vi "ErrorLoop.vi"(8 "Error In":errorcluster, 11 "Message Queues":T1) -> (0 "Error Out":errorcluster)   [LabVIEW 2017, in "Client.lvlib" / "ClientErrorHandler.lvlib"]
doc: "This Loop receives all errors and warnings coming from any other loop. It then validates if the error is critical, and if yes, it stops the Application by sending a UserEvent to the EHL.\nThis Loop also logs all Errors to a textfile."
uses:
  ClientErrorHandler.lvlib
  Error Cluster From Error Code.vi
  Error Ring.xnode
  Message Queue.lvlib
  ClientLogger.lvlib
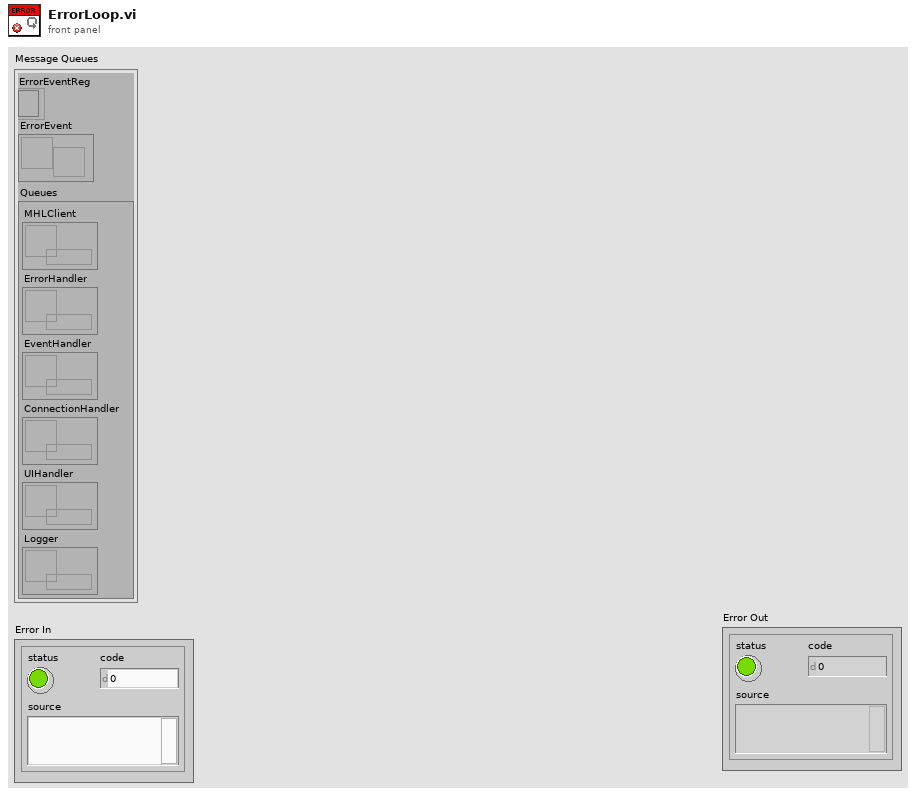
[diagram p1: front panel]
types:
  T1 = cluster{"ErrorEventReg":refnum<event-registration>, "ErrorEvent":refnum<user-event>, "Queues":cluster{"MHLClient":refnum<queue>, "ErrorHandler":refnum<queue>, "EventHandler":refnum<queue>, "ConnectionHandler":refnum<queue>, "UIHandler":refnum<queue>, "Logger":refnum<queue>}}
  T2 = cluster{"ErrorLoopInitData":cluster{"ErrorsToIgnore":i32[]}}
  T3 = cluster{"ClientTimeout (s)":u32, "LogPath":path, "ErrorsToIgnore":i32[], "OracleData":cluster{"DBname":string, "User":string, "Password":string}}
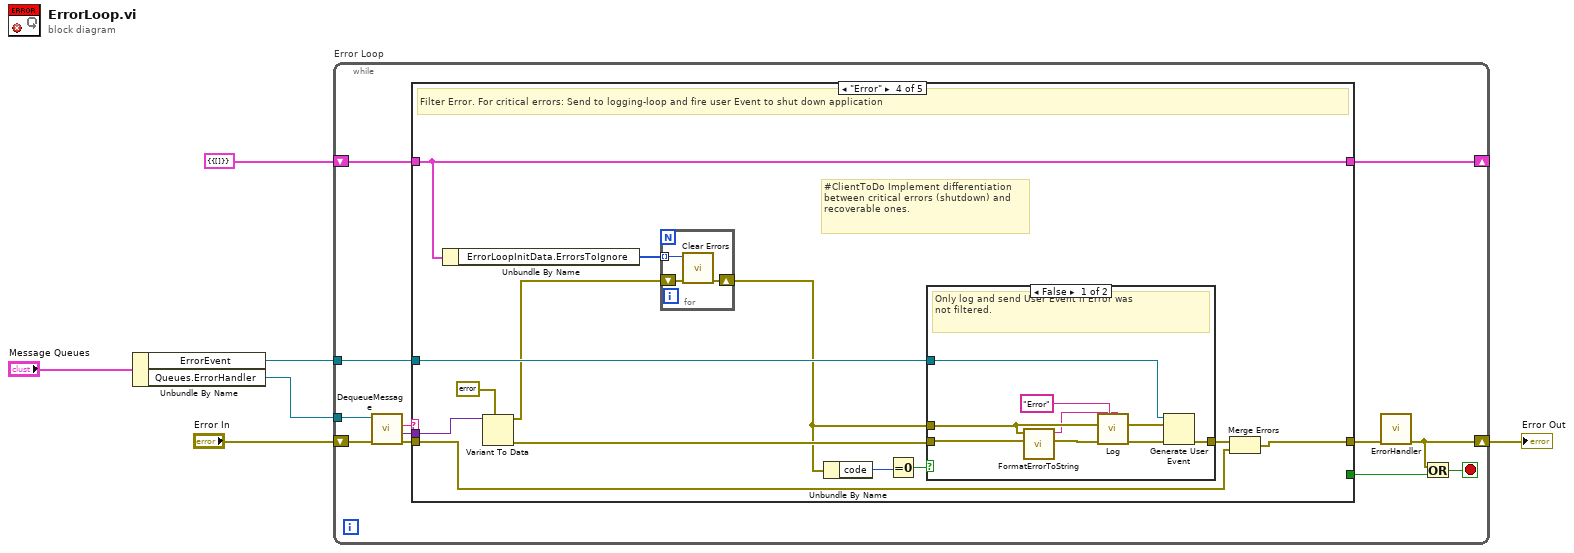
[diagram p0: block diagram]
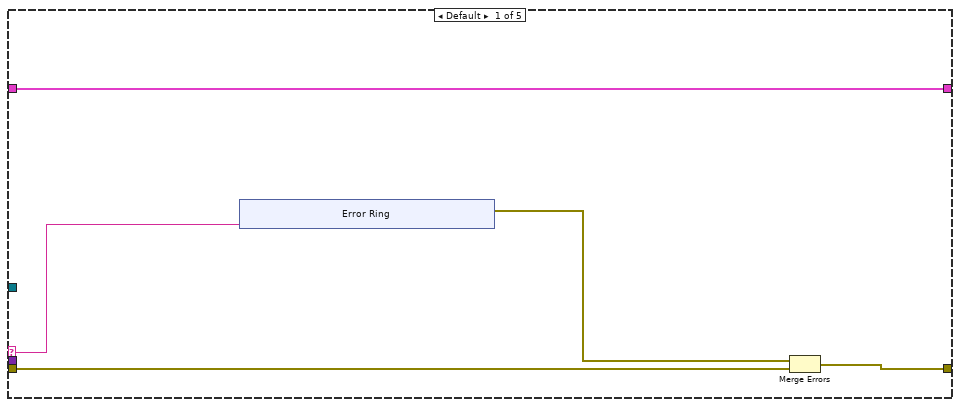
[diagram p2: hidden frame]
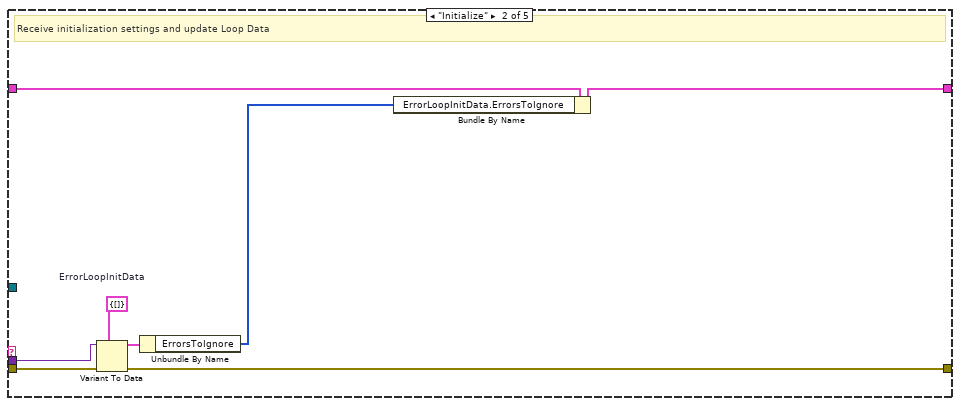
[diagram p3: hidden frame]
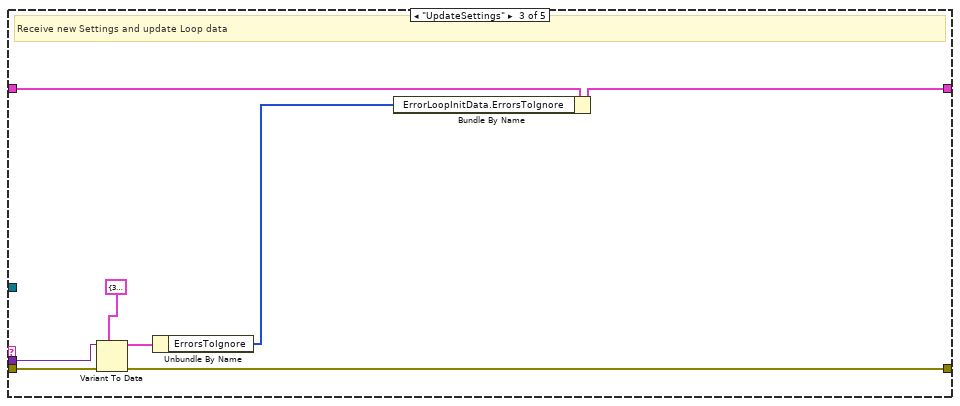
[diagram p4: hidden frame]
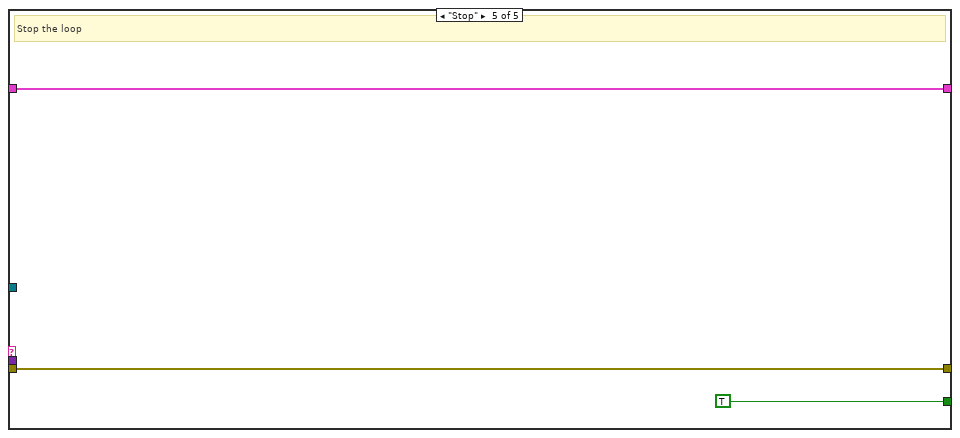
[diagram p6: hidden frame]
diagram:
  n1 = Unbundle By Name("Message Queues") -> ("ErrorEvent"=w3:refnum<user-event>, "Queues.ErrorHandler"=w4:refnum<queue>)
  n2 = while "Error Loop" {
    shift-right: [w7] -> w5
    shift-left: "Error In" -> [w18]
    tunnel: w4 -> [w16]
    tunnel: w3 -> [w11]
    shift-right: [w9] -> _
    shift-left: T2 {"ErrorLoopInitData"={"ErrorsToIgnore"=[]}} ("ErrorLoopData") -> [w10]
    stop <- w8 stop-if-true
    n3 = call "DequeueMessage.vi"("error in (no error)"=w18, "Message Queue"=w16) -> ("error out"=w17:errorcluster, "Message Data"=w14:variant, "Message"=w15:string)  [unwired: 5 in, 2 out]
    n4 = case shown="\"Error\"" w15 {
      selector: w15 -> [w20 _ _ _ _]
      tunnel: [w22 w37 w45 w55 w74] -> w12
      tunnel: w17 -> [w23 w38 w46 w53 w74]
      tunnel: w14 -> [_ w36 w44 w57 _]
      tunnel: [_ _ _ _ TRUE] -> w13
      tunnel: w11 -> [_ _ _ w58 _]
      tunnel: w10 -> [w19 w35 w42 w48 w72]
      tunnel: [w19 w34 w41 w48 w72] -> w9
      frame Default {
        n5 = xnode "Error Ring"("parameter 0"=w20) -> ("error out"=w21:errorcluster)
        n6 = Merge Errors(w21, w23) -> (w22:errorcluster)
      }
      frame "Initialize" {
        w33 = cluster{"ErrorsToIgnore":i32[]} {"ErrorsToIgnore"=[]}  # ErrorLoopInitData
        # "Receive initialization settings and update Loop Data"
        n7 = Variant To Data(error in=w38, type=w33, Variant=w36) -> (data=w32:cluster{"ErrorsToIgnore":i32[]}, error out=w37:errorcluster)
        n8 = Unbundle By Name(w32) -> ("ErrorsToIgnore"=w31:i32[])
        n9 = Bundle By Name(cluster=w35, "ErrorLoopInitData.ErrorsToIgnore"=w31) -> (w34:T2)
      }
      frame "UpdateSettings" {
        # "Receive new Settings and update Loop data"
        n10 = Variant To Data(error in=w46, type=T3 {"ClientTimeout (s)"=30, "LogPath"=path "C:/Users/jgoebel/Documents/GitHub/AEDashboard/ServerLib/Data/ServerLog.tdms", "ErrorsToIgnore"=[], "OracleData"={"DBname"="", "User"="", "Password"=""}} ("ServerINI"), Variant=w44) -> (data=w40:T3, error out=w45:errorcluster)
        n11 = Unbundle By Name(w40) -> ("ErrorsToIgnore"=w39:i32[])
        n12 = Bundle By Name(cluster=w42, "ErrorLoopInitData.ErrorsToIgnore"=w39) -> (w41:T2)
      }
      frame "Error" {
        # "#ClientToDo Implement differentiation between critical errors (shutdown) and recoverable ones."
        # "Filter Error. For critical errors: Send to logging-loop and fire user Event to shut down application"
        n13 = Unbundle By Name(w48) -> ("ErrorLoopInitData.ErrorsToIgnore"=w47:i32[])
        n14 = Variant To Data(type=errorcluster {"status"=FALSE, "code"=0, "source"=""} ("error constant"), Variant=w57) -> (data=w52:errorcluster, error out=w54:errorcluster)  [unwired: 1 in]
        n15 = for {
          shift-right: [w70] -> w51
          shift-left: w52 -> [w71]
          tunnel: w47 -> [w69] mode=indexing
          n16 = call "Clear Errors.vi"("error in (no error)"=w71, "specific error code to clear (0: all)"=w69) -> ("error out"=w70:errorcluster)  [unwired: 4 in, 1 out]
        }
        n17 = Unbundle By Name(w51) -> ("code"=w50:i32)
        n18 = Equal To 0?(x=w50) -> (x = 0?=w49:bool)
        n19 = case shown="False" w49 {
          tunnel: [w66 w68] -> w59
          tunnel: w58 -> [w64 _]
          tunnel: w54 -> [w65 w68]
          tunnel: w51 -> [w67 _]
          frame False {
            # "Only log and send User Event if Error was\nnot filtered."
            n20 = call "FormatErrorToString.vi"("error in"=w65, "ErrorToLog"=w67) -> ("error out"=w61:errorcluster, "ErrorString"=w62:string)  [unwired: 8 in]
            n21 = call "Log.vi"("LogMessage"=w62, "Type"="Error", "Error In"=w61) -> ("Error Out"=w60:errorcluster)  [unwired: 8 in]
            n22 = Generate User Event(user event=w64, event data cluster=w67, error in=w60) -> (error out=w66:errorcluster)  [unwired: 1 in, 1 out]
          }
          frame True {
            # "Error was filtered -> do nothing"
          }
        }
        n23 = Merge Errors(w59, w53) -> (w55:errorcluster)
      }
      frame "Stop" {
        # "Stop the loop"
      }
    }
    n24 = call "ErrorHandler.vi"("error in (no error)"=w12) -> ("error out"=w7:errorcluster)  [unwired: 10 in]
    n25 = Or(x=w7, y=w13) -> (x .or. y?=w8:bool)
  }
  "Error Out" <- w5
